vi "LIN_Launcher.vi"() -> ()   [LabVIEW 2014]
uses:
  <vilib>/Utility/miscctls.llb/LVPointTypeDef.ctl
  <vilib>/Utility/miscctls.llb/LVPositionTypeDef.ctl
  Typedef/TSLIN_Launcher_Data.ctl
  Typedef/TLibLIN.ctl
  Utilities/Typedef/Hardware_Subtype.ctl
  Typedef/TSLIN_SetData.ctl
  Typedef/TSLIN_SendHead.ctl
  Typedef/TSLIN_Config.ctl
  Typedef/TSLIN_Data.ctl
  Typedef/TSLIN_Transmit.ctl
  Typedef/TSLIN_LIN Schedule_Table.ctl
  Typedef/TSLIN_LIN_Set.ctl
  All_Control/Typedef/Hardware Type.ctl
  All_Control/Typedef/Blf_Log.ctl
  DataBase/Typedef/DataBase_array_index.ctl
panel:
  in  "Sender":string="LIN_Launcher"
  in  "Config":bool
  in  "Device Open":u16(ring)=1 items=["1 Device"=1, "2 Devices"=2, "3 Devices"=3, "4 Devices"=4, "5 Devices"=5, "6 Devices"=6, "7 Devices"=7, "8 Devices"=8, "9 Devices"=9, "10 Devices"=10, "11 Devices"=11, "12 Devices"=12, "13 Devices"=13, "14 Devices"=14, "15 Devices"=15, "16 Devices"=16]
  in  "DLL_PATH":path
  in  "选项卡控件":T1(tab)
  in  "STOP":bool
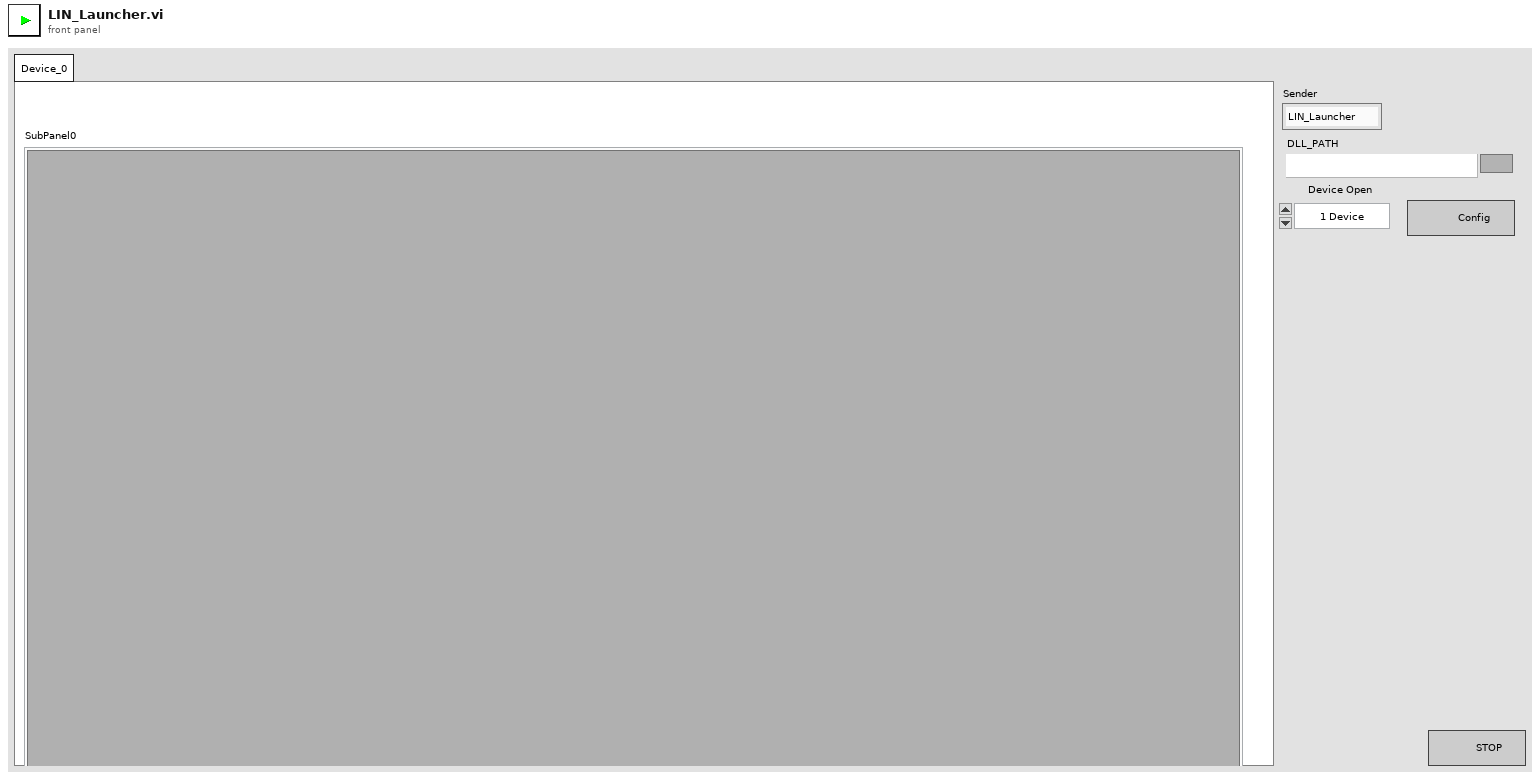
[diagram p1: front panel]
types:
  T1 = enum32{"Device_0", "Device_1", "Device_2", "Device_3", "Device_4", "Device_5", "Device_6", "Device_7", "Device_8", "Device_9", "Device_10", "Device_11", "Device_12", "Device_13", "Device_14", "Device_15"}
  T2 = typedef "LVPointTypeDef.ctl" = cluster{"Horizontal":i16, "Vertical":i16}
  T3 = typedef "LVPositionTypeDef.ctl" = cluster{"Left":i32, "Top":i32}
  T4 = typedef "TSLIN_Launcher_Data.ctl" = cluster{"DLL_PATH":path, "Channels used":u16, "Communication message":cluster{"Sender":string, "receiver":string, "message":string, "data":variant}, "error out":errorcluster}
  T5 = cluster{"Sender":string, "receiver":string, "message":string, "data":variant}
  T6 = typedef "TSLIN_Data.ctl" = cluster{"Communication message":cluster{"Sender":string, "receiver":string, "message":string, "data":variant}, "LIN_Data":T7, "LIN Data array":T16[], "error in":errorcluster, "REC_Channel":i32, "AsynCall?":bool, "DataBase_array":T17}
  T7 = typedef "TSLIN_Config.ctl" = cluster{"DLL_PATH":path, "Channels used":u16, "Funtiontype":i32, "Rx/TX":enum16{"Rx", "Tx"}, "Read message type":enum16{"Only read received messages", "Receive&send messages"}, "async&sync":enum16{"async", "sync"}, "sync_sendTimeout":u16, "LIN_SendHead":T8, "LIN_Set":T9, "LIN_DATA":cluster{"Data0":u8, "Data1":u8, "Data2":u8, "Data3":u8, "Data4":u8, "Data5":u8, "Data6":u8, "Data7":u8}, "LIN_Set_Array":T12[], "LDF":cluster{"LDF Path":path, "LDF loading channel":i32}, "Blf_Log":T13, "LIN Scheduling Table Array":T14[], "REC_Channel":i32}
  T8 = typedef "TSLIN_SendHead.ctl" = cluster{"ALINIdxchn":u8, "ALINId":u32, "ALINDLC":u32}
  T9 = typedef "TSLIN_SetData.ctl" = cluster{"Hardware Type":T10, "Hardware Subtype":T11, "AHwChannel":i32, "AAppChannel":i32, "ABaudrateKbps":sgl, "AProtocol":i32, "AldHW":i32}
  T10 = typedef "Hardware Type.ctl" = i32
  T11 = typedef "Hardware_Subtype.ctl" = enum16{"TS_UNKNOWN_DEVICE", "TSCAN_PRO", "TSCAN_Lite1", "TC1001", "TL1001", "TC1011", "TM5011", "TC1002", "TC1014", "TSCANFD2517", "TC1026", "TC1016", "TC1012", "TC1013", "TLog1002", "TC1034", "TC1018", "GW2116", "TC2115", "MP1013", "TC1113", "TC1114", "TP1013", "TC1017", "TP1018", "TF10XX", "TL1004_FD_4_LIN_2", "TE1051", "TP1051", "TP1034", "TTS9015", "TP1026", "TTS1026", "TTS1034", "TTS1018", "TL1011", "TTS1015_LiAuto", "TTS1013_LiAuto", "TTS1016Pro", "TC1054Pro", "TC1054", "TLog1038", "TO1013", "TC1034Pro", "TC1018Pro", "TC1038Pro", "TS_DEV_END"}
  T12 = typedef "TSLIN_LIN_Set.ctl" = cluster{"Set":T9, "Set_node_funtiontype":i32}
  T13 = typedef "Blf_Log.ctl" = cluster{"Blf_Log_PATH":path}
  T14 = typedef "TSLIN_LIN Schedule_Table.ctl" = cluster{"LIN_Transmit":T15, "Delay(ms)":i32}
  T15 = typedef "TSLIN_Transmit.ctl" = cluster{"Channel":i32, "Rx/TX":enum16{"Rx", "Tx"}, "Set_node_funtiontype":i32, "DLC":u32, "ID":u32, "FDatas":cluster{"value0":u8, "value 1":u8, "value 2":u8, "value 3":u8, "value 4":u8, "value 5":u8, "value 6":u8, "value 7":u8}}
  T16 = typedef "TLibLIN.ctl" = cluster{"Ch":u8, "Code":u8, "Properties":u8, "FDLC":u8, "ID":u8, "Checksum":u8, "FStaus":u8, "FTimeUS":u64, "FDatas":cluster{"value0":u8, "value 1":u8, "value 2":u8, "value 3":u8, "value 4":u8, "value 5":u8, "value 6":u8, "value 7":u8}}
  T17 = typedef "DataBase_array_index.ctl" = refnum<vi>
  T18 = enum32{"invalid app kind", "Development System", "Run Time System", "Student Edition", "Embedded LabVIEW", "Evaluation", "Custom"}
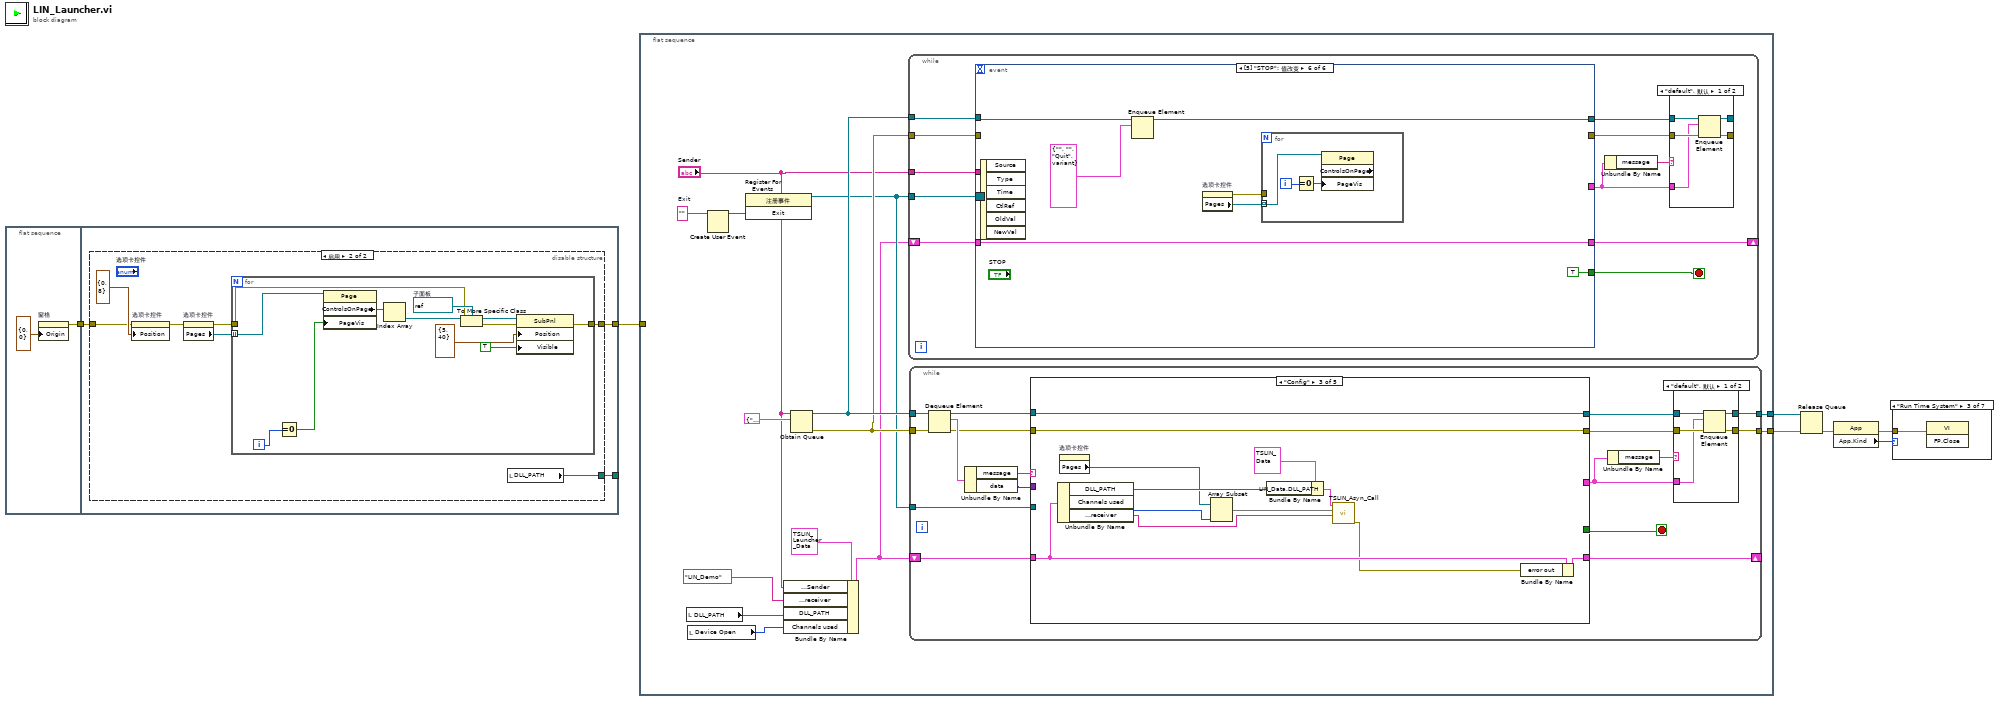
[diagram p0: block diagram]
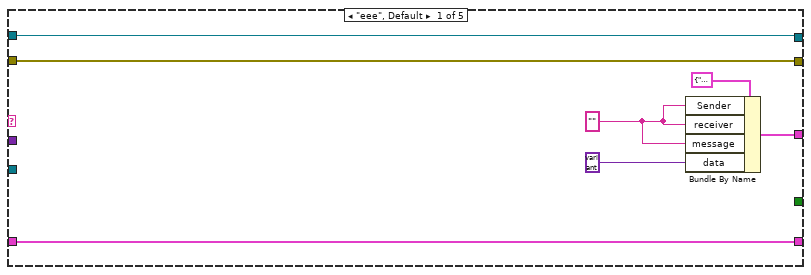
[diagram p3: hidden frame]
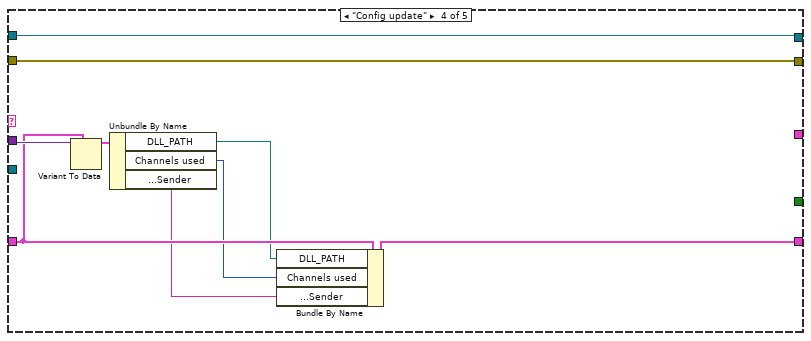
[diagram p5: hidden frame]
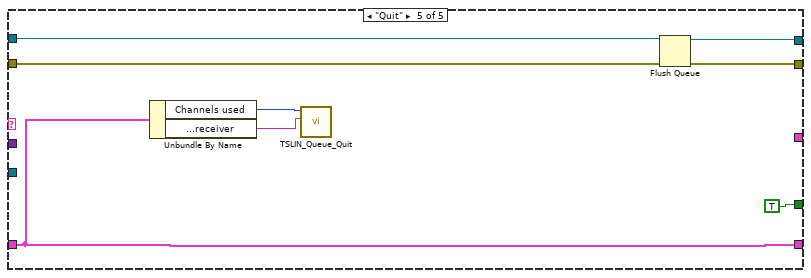
[diagram p6: hidden frame]
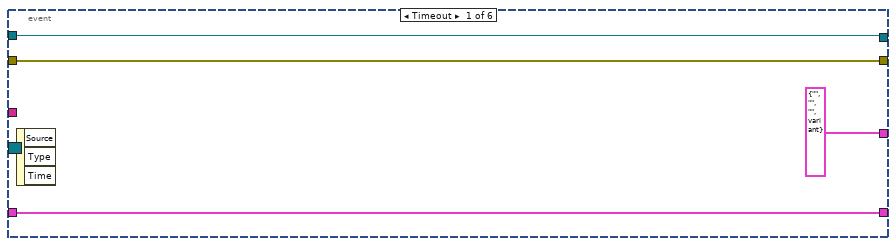
[diagram p8: hidden frame]
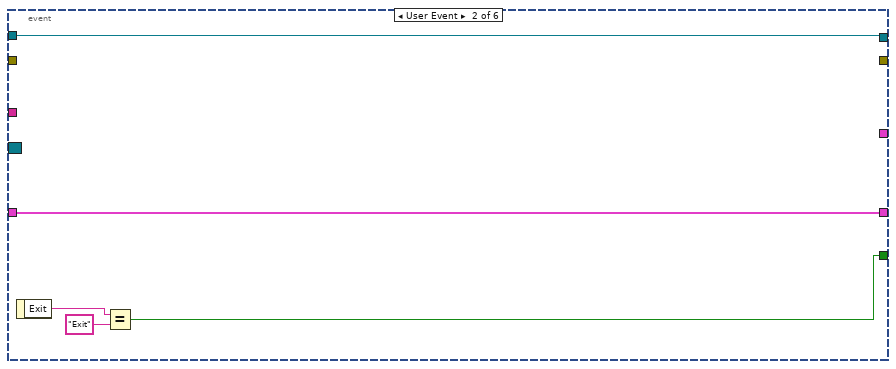
[diagram p9: hidden frame]
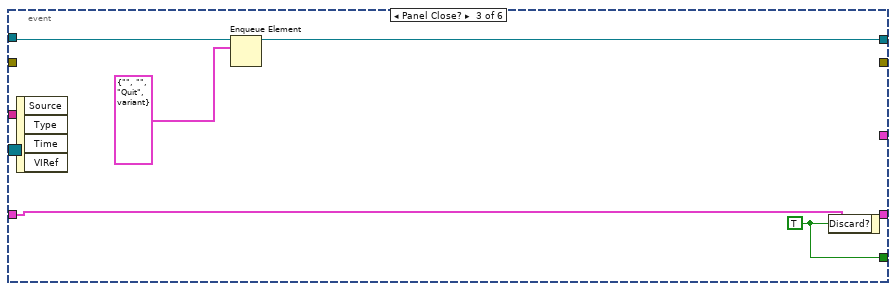
[diagram p10: hidden frame]
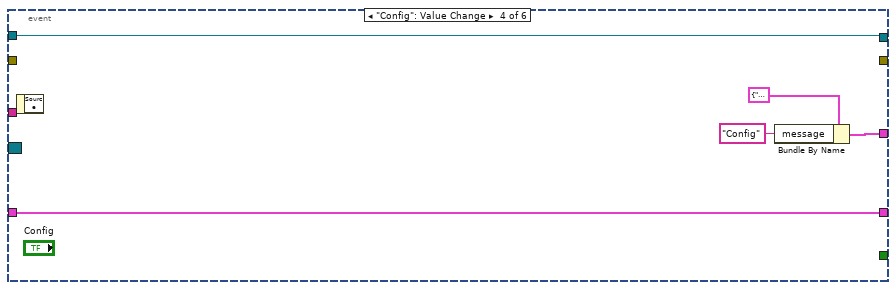
[diagram p11: hidden frame]
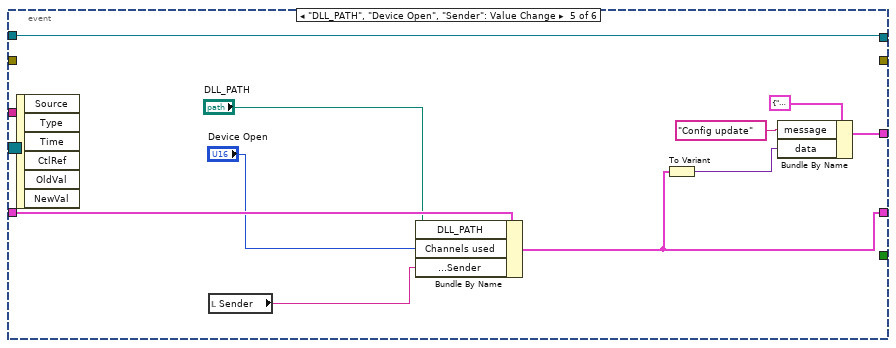
[diagram p12: hidden frame]
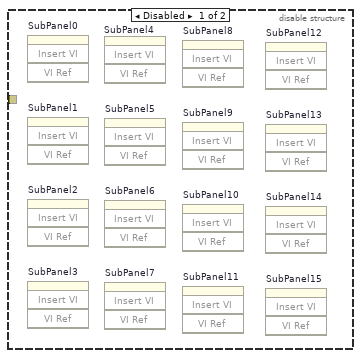
[diagram p19: hidden frame]
diagram:
  n1 = flat-sequence {
    tunnel: [w8] -> w7
    tunnel: w7 -> [w12]
    tunnel: [w11] -> w1
    tunnel: [w10] -> _
    frame #0 {
      n2 = property on="窗格" class="Pane"("Origin"=T2 {"Horizontal"=0, "Vertical"=0} ("原点")) -> (error out=w8:errorcluster)  [unwired: 2 in, 1 out]
    }
    frame #1 {
      n3 = disable-structure shown="启用" {
        disable-tunnel: w12 -> [_ w17]
        disable-tunnel: [_ w14] -> w11
        disable-tunnel: [_ w13] -> w10
        frame Disabled {
          n4 = invoke on="SubPanel0" class="SubPnl" method="Insert VI"() -> ()  [unwired: 4 in, 4 out]
          n5 = invoke on="SubPanel1" class="SubPnl" method="Insert VI"() -> ()  [unwired: 4 in, 4 out]
          n6 = invoke on="SubPanel2" class="SubPnl" method="Insert VI"() -> ()  [unwired: 4 in, 4 out]
          n7 = invoke on="SubPanel3" class="SubPnl" method="Insert VI"() -> ()  [unwired: 4 in, 4 out]
          n8 = invoke on="SubPanel4" class="SubPnl" method="Insert VI"() -> ()  [unwired: 4 in, 4 out]
          n9 = invoke on="SubPanel5" class="SubPnl" method="Insert VI"() -> ()  [unwired: 4 in, 4 out]
          n10 = invoke on="SubPanel6" class="SubPnl" method="Insert VI"() -> ()  [unwired: 4 in, 4 out]
          n11 = invoke on="SubPanel7" class="SubPnl" method="Insert VI"() -> ()  [unwired: 4 in, 4 out]
          n12 = invoke on="SubPanel8" class="SubPnl" method="Insert VI"() -> ()  [unwired: 4 in, 4 out]
          n13 = invoke on="SubPanel9" class="SubPnl" method="Insert VI"() -> ()  [unwired: 4 in, 4 out]
          n14 = invoke on="SubPanel10" class="SubPnl" method="Insert VI"() -> ()  [unwired: 4 in, 4 out]
          n15 = invoke on="SubPanel11" class="SubPnl" method="Insert VI"() -> ()  [unwired: 4 in, 4 out]
          n16 = invoke on="SubPanel12" class="SubPnl" method="Insert VI"() -> ()  [unwired: 4 in, 4 out]
          n17 = invoke on="SubPanel13" class="SubPnl" method="Insert VI"() -> ()  [unwired: 4 in, 4 out]
          n18 = invoke on="SubPanel14" class="SubPnl" method="Insert VI"() -> ()  [unwired: 4 in, 4 out]
          n19 = invoke on="SubPanel15" class="SubPnl" method="Insert VI"() -> ()  [unwired: 4 in, 4 out]
        }
        frame Enabled {
          n20 = property on="选项卡控件" class="TabCtl (严格)"(error in=w17, "Position"=T3 {"Left"=0, "Top"=8} ("位置")) -> (error out=w16:errorcluster)  [unwired: 1 in, 1 out]
          n21 = property on="选项卡控件" class="TabCtl (严格)"(error in=w16) -> (error out=w15:errorcluster, "Pages"=w19:refnum<vi>[])  [unwired: 1 in, 1 out]
          n22 = for {
            tunnel: w19 -> [w31] mode=indexing
            tunnel: w15 -> [w24]
            tunnel: [w23] -> w14
            i -> [w21]
            w28 = refnum<vi> refnum  # 子面板
            n23 = Equal To 0?(x=w21) -> (x = 0?=w20:bool)
            n24 = property class="Page"(reference=w31, "PageVis"=w20) -> ("ControlsOnPage"=w30:refnum<vi>[])  [unwired: 1 in, 2 out]
            n25 = Index Array(array=w30) -> (element=w29:refnum<vi>)  [unwired: 1 in]
            n26 = To More Specific Class(target class=w28, reference=w29, error in=w24) -> (specific class reference=w27:refnum<vi>, error out=w26:errorcluster)
            n27 = property class="SubPnl"(reference=w27, error in=w26, "Position"=T3 {"Left"=5, "Top"=40} ("位置"), "Visible"=TRUE ("可见")) -> (error out=w23:errorcluster)  [unwired: 1 out]
          }
          n28 = local read "DLL_PATH"() -> (w13:path)
        }
      }
    }
  }
  n29 = flat-sequence {
    tunnel: [w44] -> w6
    tunnel: [w43] -> w5
    tunnel: w1 -> [_]
    frame #0 {
      w37 = ""  # Exit
      n30 = local read "DLL_PATH"() -> (w33:path)
      n31 = local read "Device Open"() -> (w32:u16)
      n32 = Create User Event(user event datatype=w37) -> (user event=w38:refnum<user-event>)  [unwired: 1 in, 1 out]
      n33 = register-events(w38) -> (reference out=w36:refnum<event-registration>)  [unwired: 2 in, 1 out]
      n34 = Bundle By Name(cluster=T4 {"DLL_PATH"=path "", "Channels used"=1, "Communication message"={"Sender"="", "receiver"="", "message"="", "data"=variant}, "error out"={"status"=FALSE, "code"=0, "source"=""}} ("Data"), "Communication message.Sender"="Sender", "Communication message.receiver"="LIN_Demo", "DLL_PATH"=w33, "Channels used"=w32) -> (w35:T4)
      n35 = Obtain Queue(name (unnamed)="Sender", element data type=T5 {"Sender"="", "receiver"="", "message"="", "data"=variant} ("Communication message")) -> (queue out=w45:refnum<queue>, error out=w41:errorcluster)  [unwired: 3 in, 1 out]
      n36 = while {
        tunnel: w45 -> [w118]
        tunnel: w41 -> [w116]
        tunnel: "Sender" -> [w112]
        tunnel: w36 -> [w111]
        shift-right: [w109] -> _
        shift-left: w35 -> [w110]
        stop <- w119 stop-if-true
        n37 = event shown="[5] \"STOP\": 值改变" {
          selector: w111 -> [_ _ _ _ _ _]
          dyn-events: _ -> [_ _ _ _ _ _]
          timeout: _ -> [_ _ _ _ _ _]
          tunnel: [_ w132 w140 _ _ TRUE ("放弃？")] -> w119
          tunnel: w118 -> [w130 w135 w139 w145 w155 w161]
          tunnel: [w130 w135 w137 w145 w155 w160] -> w117
          tunnel: [T5 {"Sender"="", "receiver"="", "message"="", "data"=variant} ("Communication message") _ _ w143 w152 _] -> w114
          tunnel: [w129 _ _ _ _ _] -> w115
          tunnel: w116 -> [w129 _ _ _ _ _]
          tunnel: w112 -> [_ _ _ _ _ _]
          tunnel: w110 -> [w127 w131 w136 w141 w154 w158]
          tunnel: [w127 w131 w136 w141 w148 w158] -> w109
          event Timeout {
            n38 = event-data() -> ()  [unwired: 1 in, 3 out]
          }
          event User Event {
            n39 = event-data() -> ("Exit"=w134:string)  [unwired: 1 in]
            n40 = Equal?(x=w134, y="Exit") -> (x = y?=w132:bool)
          }
          event Panel Close? {
            w140 = TRUE ("放弃？")
            n41 = event-data() -> ()  [unwired: 1 in, 4 out]
            n42 = Enqueue Element(queue=w139, element=T5 {"Sender"="", "receiver"="", "message"="Quit", "data"=variant} ("Communication message")) -> (queue out=w137:refnum<queue>)  [unwired: 2 in, 2 out]
            n43 = event-data("Discard?"=w140) -> ()  [unwired: 1 in, 1 out]
          }
          event "Config": Value Change {
            n44 = event-data() -> ()  [unwired: 1 in, 1 out]
            n45 = Bundle By Name(cluster=T5 {"Sender"="", "receiver"="", "message"="", "data"=variant} ("Communication message"), "message"="Config") -> (w143:T5)
          }
          event "DLL_PATH", "Device Open", "Sender": Value Change {
            n46 = event-data() -> ()  [unwired: 1 in, 6 out]
            n47 = local read "Sender"() -> (w146:string)
            n48 = Bundle By Name(cluster=w154, "DLL_PATH"="DLL_PATH", "Channels used"="Device Open", "Communication message.Sender"=w146) -> (w148:T4)
            n49 = To Variant(anything=w148) -> (Variant=w147:variant)
            n50 = Bundle By Name(cluster=T5 {"Sender"="", "receiver"="", "message"="", "data"=variant} ("Communication message"), "message"="Config update", "data"=w147) -> (w152:T5)
          }
          event "STOP": Value Change {
            n51 = event-data() -> ()  [unwired: 1 in, 6 out]
            n52 = Enqueue Element(queue=w161, element=T5 {"Sender"="", "receiver"="", "message"="Quit", "data"=variant} ("Communication message")) -> (queue out=w160:refnum<queue>)  [unwired: 2 in, 2 out]
            n53 = property on="选项卡控件" class="TabCtl (严格)"() -> (error out=w156:errorcluster, "Pages"=w157:refnum<vi>[])  [unwired: 2 in, 1 out]
            n54 = for {
              tunnel: w157 -> [w165] mode=indexing
              tunnel: w156 -> [_]
              i -> [w164]
              n55 = Equal To 0?(x=w164) -> (x = 0?=w163:bool)
              n56 = property class="Page" props=["ControlsOnPage", "PageVis"](reference=w165, "PageVis"=w163) -> ()  [unwired: 1 in, 3 out]
            }
          }
        }
        n57 = Unbundle By Name(w114) -> ("message"=w113:string)
        n58 = case shown="\"default\", 默认" w113 {
          tunnel: w117 -> [w124 w126]
          tunnel: w115 -> [w123 w125]
          tunnel: w114 -> [w122 _]
          tunnel: [w121 w126] -> _
          tunnel: [w120 w125] -> _
          frame "default", Default {
            n59 = Enqueue Element(queue=w124, element=w122, error in (no error)=w123) -> (queue out=w121:refnum<queue>, error out=w120:errorcluster)  [unwired: 1 in, 1 out]
          }
          frame "" {
          }
        }
      }
      n60 = while {
        tunnel: w45 -> [w62]
        tunnel: w41 -> [w61]
        tunnel: [w53] -> w44
        tunnel: [w52] -> w43
        shift-right: [w47] -> _
        shift-left: w35 -> [w48]
        tunnel: w36 -> [w46]
        stop <- w51 stop-if-true
        n61 = Dequeue Element(queue=w62, error in (no error)=w61) -> (queue out=w58:refnum<queue>, element=w60:T5, error out=w57:errorcluster)  [unwired: 1 in, 1 out]
        n62 = Unbundle By Name(w60) -> ("message"=w59:string, "data"=w54:variant)
        n63 = case shown="\"Config\"" w59 {
          tunnel: [w76 w79 w91 w100 w107] -> w56
          tunnel: w58 -> [w76 w79 w91 w100 w106]
          tunnel: w57 -> [w75 w78 w90 w99 w104]
          tunnel: [w75 w78 w90 w99 w105] -> w55
          tunnel: w54 -> [_ _ _ w98 _]
          tunnel: [_ _ _ _ TRUE] -> w51
          tunnel: [w73 _ _ _ _] -> w50
          tunnel: [w70 w77 w89 w96 w103] -> w47
          tunnel: w48 -> [w70 w77 w88 w97 w103]
          tunnel: w46 -> [_ _ _ _ _]
          frame "eee", Default {
            w71 = ""
            n64 = Bundle By Name(cluster=T5 {"Sender"="", "receiver"="", "message"="", "data"=variant} ("Communication message"), "Sender"=w71, "receiver"=w71, "message"=w71, "data"=variant) -> (w73:T5)
          }
          frame "Init" {
          }
          frame "Config" {
            n65 = Unbundle By Name(w88) -> ("DLL_PATH"=w87:path, "Channels used"=w84:u16, "Communication message.receiver"=w86:string)
            n66 = property on="选项卡控件" class="TabCtl (严格)"() -> ("Pages"=w83:refnum<vi>[])  [unwired: 2 in, 2 out]
            n67 = Array Subset(array=w83, length=w84) -> (w80:refnum<vi>[])  [unwired: 1 in]
            n68 = Bundle By Name(cluster=T6 {"Communication message"={"Sender"="", "receiver"="", "message"="", "data"=variant}, "LIN_Data"={"DLL_PATH"=path "", "Channels used"=1, "Funtiontype"=0, "Rx/TX"=enum."Rx", "Read message type"=enum."Receive&send messages", "async&sync"=enum."async", "sync_sendTimeout"=0, "LIN_SendHead"={"ALINIdxchn"=0, "ALINId"=0, "ALINDLC"=0}, "LIN_Set"={"Hardware Type"=2, "Hardware Subtype"=enum."TC1016", "AHwChannel"=0, "AAppChannel"=19, "ABaudrateKbps"=19.2, "AProtocol"=2, "AldHW"=0}, "LIN_DATA"={"Data0"=0, "Data1"=0, "Data2"=0, "Data3"=0, "Data4"=0, "Data5"=0, "Data6"=0, "Data7"=0}, "LIN_Set_Array"=[], "LDF"={"LDF Path"=path "", "LDF loading channel"=0}, "Blf_Log"={"Blf_Log_PATH"=path ""}, "LIN Scheduling Table Array"=[], "REC_Channel"=0}, "LIN Data array"=[], "error in"={"status"=FALSE, "code"=0, "source"=""}, "REC_Channel"=0, "AsynCall?"=FALSE, "DataBase_array"=refnum} ("Data"), "LIN_Data.DLL_PATH"=w87) -> (w81:T6)
            n69 = call "TSLIN_Asyn_Call.vi"("Queue Name"=w86, "Ref_Arry"=w80, "Data"=w81) -> ("error out"=w85:errorcluster)  [unwired: 8 in]
            n70 = Bundle By Name(cluster=w88, "error out"=w85) -> (w89:T4)
          }
          frame "Config update" {
            n71 = Variant To Data(type=w97, Variant=w98) -> (data=w95:T4)  [unwired: 1 in, 1 out]
            n72 = Unbundle By Name(w95) -> ("DLL_PATH"=w94:path, "Channels used"=w93:u16, "Communication message.Sender"=w92:string)
            n73 = Bundle By Name(cluster=w97, "DLL_PATH"=w94, "Channels used"=w93, "Communication message.Sender"=w92) -> (w96:T4)
          }
          frame "Quit" {
            n74 = Unbundle By Name(w103) -> ("Channels used"=w102:u16, "Communication message.receiver"=w101:string)
            n75 = call "TSLIN_Queue_Quit.vi"("receiver"=w101, "Channels used"=w102) -> ()  [unwired: 9 in, 1 out]
            n76 = Flush Queue(queue=w106, error in (no error)=w104) -> (queue out=w107:refnum<queue>, error out=w105:errorcluster)  [unwired: 1 out]
          }
        }
        n77 = Unbundle By Name(w50) -> ("message"=w49:string)
        n78 = case shown="\"default\", 默认" w49 {
          tunnel: w56 -> [w67 w69]
          tunnel: w55 -> [w66 w68]
          tunnel: w50 -> [w65 _]
          tunnel: [w64 w69] -> w53
          tunnel: [w63 w68] -> w52
          frame "default", Default {
            n79 = Enqueue Element(queue=w67, element=w65, error in (no error)=w66) -> (queue out=w64:refnum<queue>, error out=w63:errorcluster)  [unwired: 1 in, 1 out]
          }
          frame "" {
          }
        }
      }
    }
  }
  n80 = Release Queue(queue=w6, error in (no error)=w5) -> (error out=w4:errorcluster)  [unwired: 1 in, 2 out]
  n81 = property class="App"(error in=w4) -> (error out=w3:errorcluster, "App.Kind"=w2:T18)  [unwired: 1 in, 1 out]
  n82 = case shown="\"Run Time System\"" w2 {
    tunnel: w3 -> [_ _ w166 _ _ _ _]
    frame "invalid app kind", Default {
    }
    frame "Development System" {
    }
    frame "Run Time System" {
      n83 = invoke class="VI" method="FP.Close"(error in=w166) -> ()  [unwired: 2 in, 3 out]
    }
    frame "Student Edition" {
    }
    frame "Embedded LabVIEW" {
    }
    frame "Evaluation" {
    }
    frame "Custom" {
    }
  }
